vi "Beep.vi"(8 "error in":errorcluster, 10 "numChunks in":i32=1, 11 "frequency in":dbl=1000.0) -> (0 "error out":errorcluster)   [LabVIEW 2010, in "Labricks.lvlib" / "Game.lvclass"]
uses:
  Game.lvclass
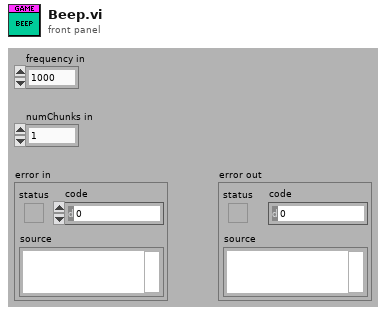
[diagram p1: front panel]
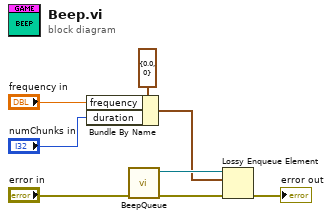
[diagram p0: block diagram]
diagram:
  n1 = Bundle By Name(cluster=cluster{"frequency":dbl, "duration":i32} {"frequency"=0.0, "duration"=0} ("BeepConfig"), "frequency"="frequency in", "duration"="numChunks in") -> (w1:cluster{"frequency":dbl, "duration":i32})
  n2 = call "BeepQueue.vi"("error in"="error in") -> ("error out"=w6:errorcluster, "queue out"=w8:refnum<queue>)  [unwired: 5 in]
  n3 = Lossy Enqueue Element(queue=w8, element=w1, error in (no error)=w6) -> (error out=→"error out":errorcluster)  [unwired: 3 out]
